vi "Locate Line Cross.vi"(7 "Tolerance":cluster{"x":dbl, "y":dbl, "a":dbl}={"x"=2.0, "y"=2.0, "a"=2.0}, 8 "error in":errorcluster, 9 "Type":string, 11 "color":string) -> (0 "error out":errorcluster, 1 "Found":bool, 2 "Range":dbl, 3 "result":T1, 4 "Close":bool, 5 "picture":picture)   [LabVIEW 2013]
uses:
  ROS/Code/SubVIs/BaxterCamera.ctl
  ROS/Code/SubVIs/BaxterSide.ctl
  <vilib>/Analysis/NI_AALBase.lvlib
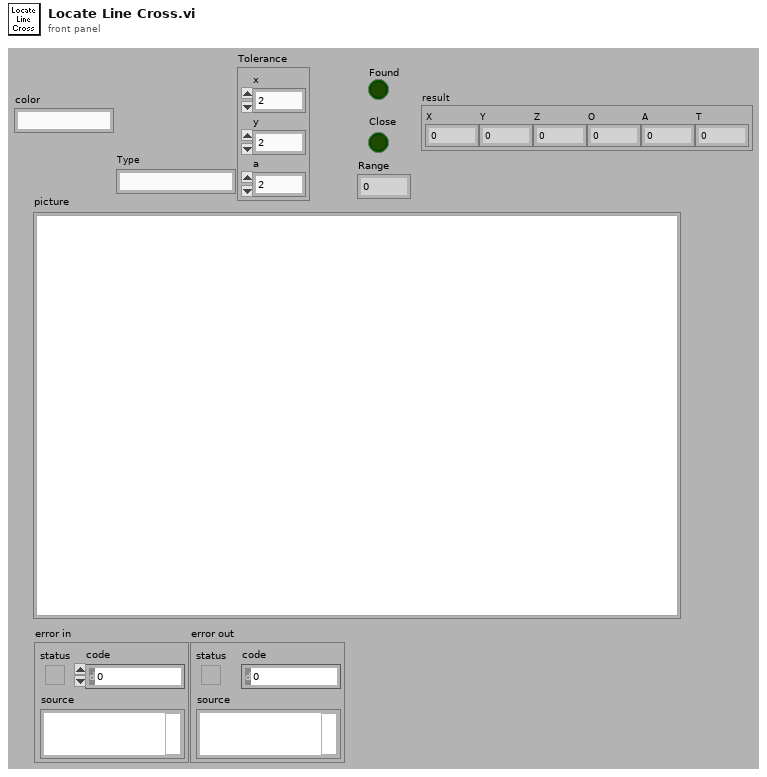
[diagram p1: front panel]
types:
  T1 = cluster{"X":dbl, "Y":dbl, "Z":dbl, "O":dbl, "A":dbl, "T":dbl}
  T2 = typedef "BaxterSide.ctl" = enum16{"left", "right"}
  T3 = typedef "BaxterCamera.ctl" = enum16{"left_hand_camera", "right_hand_camera", "head_camera"}
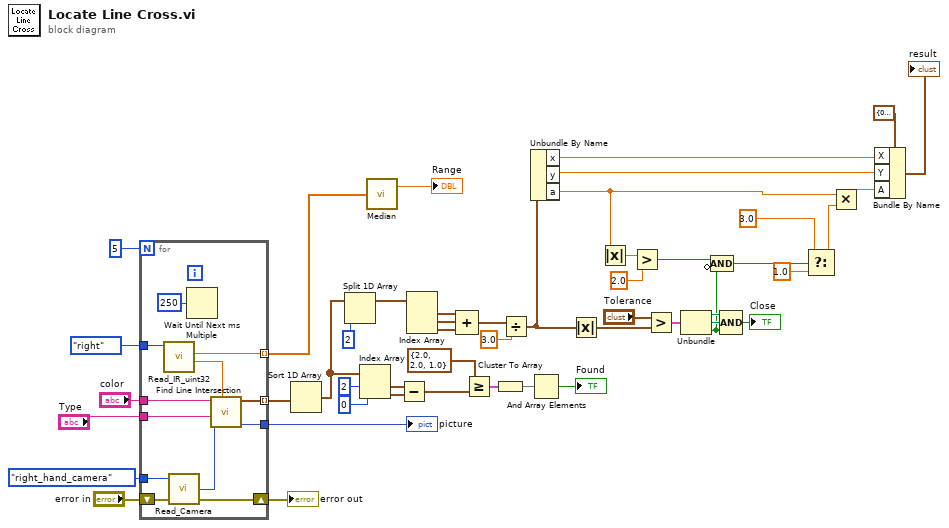
[diagram p0: block diagram]
diagram:
  n1 = for {
    N: 5 -> [_]
    tunnel: [w61] -> w49
    shift-right: [w57] -> w48
    shift-left: "error in" -> [w58]
    tunnel: [w56] -> w46 mode=indexing
    tunnel: [w54] -> w22 mode=indexing
    tunnel: "color" -> [w53]
    tunnel: BaxterCamera."right_hand_camera" ("Camera") -> [w52]
    tunnel: BaxterSide."right" ("Side") -> [w51]
    tunnel: "Type" -> [w50]
    n2 = call "Read_IR_uint32.vi"("Side"=w51) -> ("mm/pixel"=w55:dbl, "Distance"=w54:dbl)  [unwired: 4 in, 2 out]
    n3 = call "Read_Camera.vi"("Camera"=w52, "error in"=w58) -> ("picture"=w59:picture, "error out"=w57:errorcluster)  [unwired: 1 in, 3 out]
    n4 = Wait Until Next ms Multiple(millisecond multiple=u32 250) -> ()  [unwired: 1 out]
    n5 = call "Find Line Intersection.vi"("mm/pixel"=w55, "picture"=w59, "Type"=w50, "Color"=w53) -> ("picture"=w61:picture, "Result"=w56:cluster{"x":dbl, "y":dbl, "a":dbl})  [unwired: 4 in, 2 out]
  }
  "picture" <- w49
  "error out" <- w48
  n6 = Sort 1D Array(array=w46) -> (sorted array=w38:cluster{"x":dbl, "y":dbl, "a":dbl}[])
  n7 = Split 1D Array(array=w38, index=2) -> (first subarray=w36:cluster{"x":dbl, "y":dbl, "a":dbl}[])  [unwired: 1 out]
  n8 = Index Array(array=w38, index #1=2 ("index"), index #2=0 ("index")) -> (element #1=w43:cluster{"x":dbl, "y":dbl, "a":dbl}, element #2=w42:cluster{"x":dbl, "y":dbl, "a":dbl})
  n9 = call <vilib>:"Median.vi"("X"=w22) -> ("median"=→"Range":dbl)  [unwired: 1 out]
  n10 = Subtract(x=w43, y=w42) -> (x-y=w41:cluster{"x":dbl, "y":dbl, "a":dbl})
  n11 = Index Array(array=w36) -> (element #1=w35:cluster{"x":dbl, "y":dbl, "a":dbl}, element #2=w34:cluster{"x":dbl, "y":dbl, "a":dbl}, element #3=w33:cluster{"x":dbl, "y":dbl, "a":dbl})  [unwired: 3 in]
  n12 = Compound Arithmetic op=ADD(w35, w34, w33) -> (w32:cluster{"x":dbl, "y":dbl, "a":dbl})
  n13 = Greater Or Equal?(x=cluster{"x":dbl, "y":dbl, "a":dbl} {"x"=2.0, "y"=2.0, "a"=1.0}, y=w41) -> (x >= y?=w40:cluster{"x":bool, "y":bool, "a":bool})
  n14 = Cluster To Array(cluster=w40) -> (array=w39:bool[])
  n15 = Divide(x=w32, y=3.0) -> (x/y=w14:cluster{"x":dbl, "y":dbl, "a":dbl})
  n16 = Unbundle By Name(w14) -> ("x"=w16:dbl, "y"=w13:dbl, "a"=w6:dbl)
  n17 = And Array Elements(Boolean array=w39) -> (logical AND=→"Found":bool)
  n18 = Absolute Value(x=w14) -> (abs(x)=w26:cluster{"x":dbl, "y":dbl, "a":dbl})
  n19 = Absolute Value(x=w6) -> (abs(x)=w10:dbl)
  n20 = Greater?(x=w10, y=2.0) -> (0:w8:bool)
  n21 = Greater?(x="Tolerance", y=w26) -> (0:w29:cluster{"x":bool, "y":bool, "a":bool})
  n22 = Unbundle(w29) -> ("x"=w28:bool, "y"=w27:bool, "a"=w7:bool)
  n23 = Compound Arithmetic op=AND(w8, invert w7) -> (w5:bool)
  n24 = Compound Arithmetic op=AND(w28, w27, w7) -> (→"Close":bool)
  n25 = Select(t=3.0 ("y"), s=w5, f=1.0) -> (s? t:f=w1:dbl)
  n26 = Multiply(x=w6, y=w1) -> (x*y=w4:dbl)
  n27 = Bundle By Name(cluster=T1 {"X"=0.0, "Y"=0.0, "Z"=0.0, "O"=0.0, "A"=0.0, "T"=0.0} ("Goal Axes"), "X"=w16, "Y"=w13, "A"=w4) -> (→"result":T1)
